vi "Format to Prometheus.vi"(8 "error in (no error)":errorcluster, 11 "Metric":refnum<data-value>) -> (0 "error out":errorcluster, 3 "Prometheus-formatted Metric":string[](array[string]))   [LabVIEW 2020, in "Metrics.lvlib" / "Metric.lvclass"]
uses:
  Metric.lvclass
  Metric.lvclass/Metric.ctl
  Read Name.vi
  Read Samples.vi
  Read Description.vi
  sample/Sample.lvclass
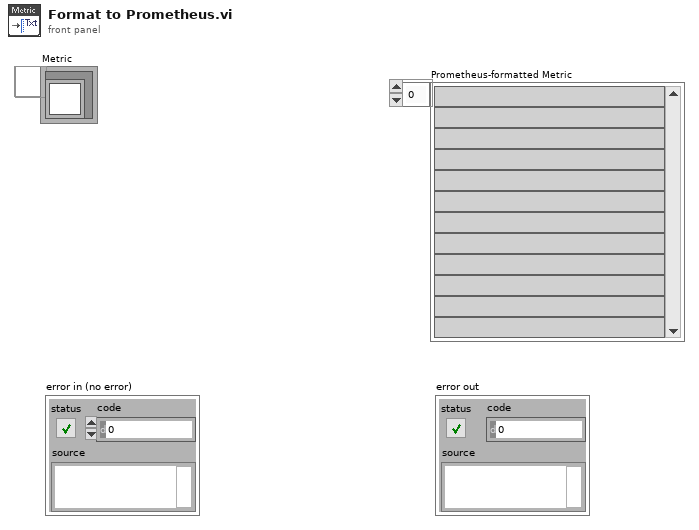
[diagram p1: front panel]
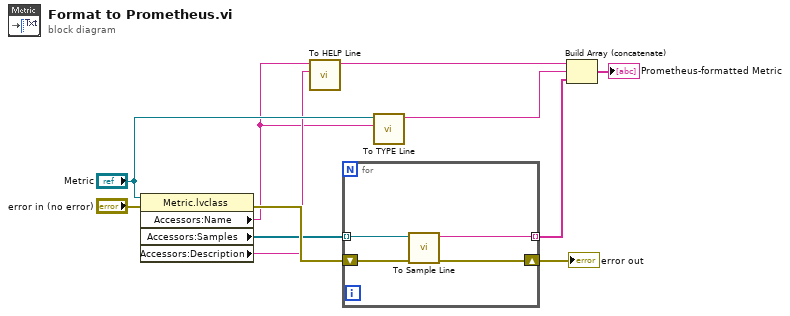
[diagram p0: block diagram]
diagram:
  n1 = property class="Metric.lvclass"(reference="Metric", error in="error in (no error)") -> (error out=w10:errorcluster, "Accessors:Name"=w5:string, "Accessors:Samples"=w8:refnum<class "Sample.lvclass">[], "Accessors:Description"=w6:string)  [unwired: 1 out]
  n2 = call "To HELP Line.vi"("Description"=w6, "Name"=w5) -> ("HELP line"=w4:string)  [unwired: 8 in, 1 out]
  n3 = for {
    tunnel: w8 -> [w15] mode=indexing
    tunnel: [w14] -> w2 mode=indexing
    shift-right: [w12] -> w11
    shift-left: w10 -> [w13]
    n4 = call "To Sample Line.vi"("error in (no error)"=w13, "Sample in"=w15) -> ("error out"=w12:errorcluster, "Sample line"=w14:string)  [unwired: 8 in]
  }
  "error out" <- w11
  n5 = call "To TYPE Line.vi"("Name"=w5, "Metric"="Metric") -> ("TYPE line"=w3:string)  [unwired: 8 in, 1 out]
  n6 = Build Array (concatenate)(w4, w3, w2) -> (→"Prometheus-formatted Metric":string[])
